vi "SMD7615 UDP Commit Move.vi"(0 "connection ID in":refnum<k16>, 1 "Acceleration":dbl, 2 "Deceleration":dbl, 5 "IP":string="192.168.1.30", 7 "Distance / Position":i32, 9 "Velocity":dbl, 11 "error in (no error)":errorcluster) -> (4 "connection ID out":refnum<k16>, 15 "error out":errorcluster)   [LabVIEW 2016, in "SMD-7615.lvlib" / "eSCL.lvlib"]
uses:
  eSCL.lvlib
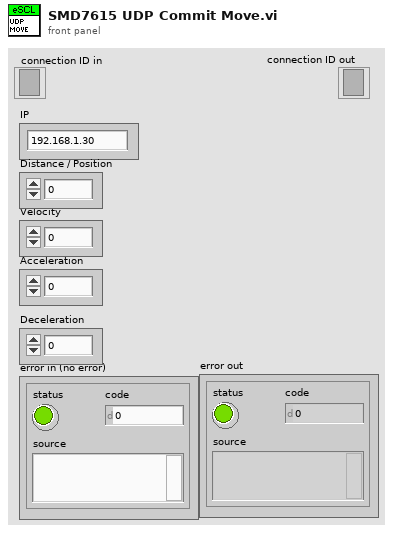
[diagram p1: front panel]
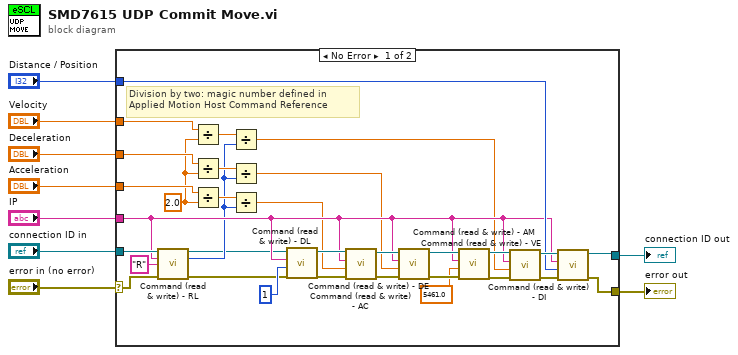
[diagram p0: block diagram]
diagram:
  n1 = case shown="No Error" "error in (no error)" {
    selector: "error in (no error)" -> [w25 w42]
    tunnel: "connection ID in" -> [w26 w43]
    tunnel: [w32 w43] -> w7
    tunnel: [w31 w42] -> w6
    tunnel: "IP" -> [w23 _]
    tunnel: "Acceleration" -> [w22 _]
    tunnel: "Deceleration" -> [w20 _]
    tunnel: "Velocity" -> [w21 _]
    tunnel: "Distance / Position" -> [w28 _]
    frame No Error {
      w19 = 2.0 ("y")
      # "Division by two: magic number defined in\nApplied Motion Host Command Reference"
      n2 = call "Command (read & write) - RL.vi"("connection ID in"=w26, "IP"=w23, "Register"="R", "error in (no error)"=w25) -> ("connection ID out"=w10:refnum<k16>, "Register Value"=w15:i32, "error out"=w11:errorcluster)  [unwired: 9 in]
      n3 = Divide(x=w21, y=w19) -> (x/y=w16:dbl)
      n4 = Divide(x=w20, y=w19) -> (x/y=w17:dbl)
      n5 = Divide(x=w22, y=w19) -> (x/y=w18:dbl)
      n6 = Divide(x=w16, y=w15) -> (x/y=w14:dbl)
      n7 = Divide(x=w17, y=w15) -> (x/y=w13:dbl)
      n8 = Divide(x=w18, y=w15) -> (x/y=w12:dbl)
      n9 = call "Command (read & write) - DL.vi"("error in (no error)"=w11, "Parameter"=1, "IP"=w23, "connection ID in"=w10) -> ("error out"=w40:errorcluster, "connection ID out"=w41:refnum<k16>)  [unwired: 5 in, 1 out]
      n10 = call "Command (read & write) - AC.vi"("error in (no error)"=w40, "Acceleration"=w12, "IP"=w23, "connection ID in"=w41) -> ("error out"=w39:errorcluster, "connection ID out"=w38:refnum<k16>)  [unwired: 5 in, 1 out]
      n11 = call "Command (read & write) - DE.vi"("error in (no error)"=w39, "Deceleration"=w13, "IP"=w23, "connection ID in"=w38) -> ("error out"=w36:errorcluster, "connection ID out"=w37:refnum<k16>)  [unwired: 5 in, 1 out]
      n12 = call "Command (read & write) - AM.vi"("error in (no error)"=w36, "Max. Acceleration"=5461.0, "IP"=w23, "connection ID in"=w37) -> ("error out"=w33:errorcluster, "connection ID out"=w34:refnum<k16>)  [unwired: 6 in]
      n13 = call "Command (read & write) - VE.vi"("error in (no error)"=w33, "Velocity"=w14, "IP"=w23, "connection ID in"=w34) -> ("error out"=w29:errorcluster, "connection ID out"=w30:refnum<k16>)  [unwired: 5 in, 1 out]
      n14 = call "Command (read & write) - DI.vi"("error in (no error)"=w29, "Distance / Position"=w28, "IP"=w23, "connection ID in"=w30) -> ("error out"=w31:errorcluster, "connection ID out"=w32:refnum<k16>)  [unwired: 5 in, 1 out]
    }
    frame Error {
    }
  }
  "connection ID out" <- w7
  "error out" <- w6
